vi "CRYCalc FSD.vi"(10 "Max Level":dbl format="%#_6p", 11 "X":dbl[](array[numeric]) format="%.2p") -> (0 "dBFSD(RMS)":dbl format="%#_6p", 1 "%FSD(RMS)":dbl format="%#_6p", 2 "dBFSD(Max)":dbl format="%#_6p", 3 "%FSD(Max)":dbl format="%#_6p")   [LabVIEW 2013]
uses:
  <vilib>/Analysis/5stat.llb/RMS (DBL).vi
  <vilib>/Analysis/NI_AALPro.lvlib
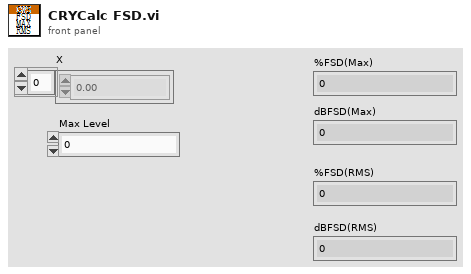
[diagram p1: front panel]
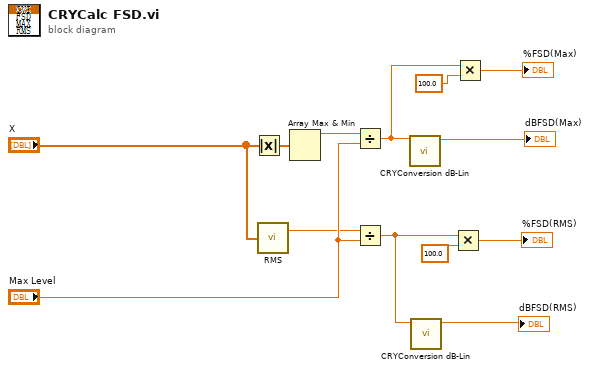
[diagram p0: block diagram]
diagram:
  n1 = Absolute Value(x="X") -> (abs(x)=w12:dbl[])
  n2 = call-poly <vilib>:"RMS.vi"("X"="X") -> ("rms value"=w3:dbl)  [unwired: 1 out]
  n3 = Array Max & Min(array=w12) -> (max value=w5:dbl)  [unwired: 3 out]
  n4 = Divide(x=w5, y="Max Level") -> (x/y=w7:dbl)
  n5 = Divide(x=w3, y="Max Level") -> (x/y=w2:dbl)
  n6 = call "CRYConversion dB-Lin.vi"("Lin In"=w7) -> ("Log Out"=→"dBFSD(Max)":dbl)  [unwired: 5 in, 3 out]
  n7 = call "CRYConversion dB-Lin.vi"("Lin In"=w2) -> ("Log Out"=→"dBFSD(RMS)":dbl)  [unwired: 5 in, 3 out]
  n8 = Multiply(x=w2, y=100.0) -> (x*y=→"%FSD(RMS)":dbl)
  n9 = Multiply(x=w7, y=100.0) -> (x*y=→"%FSD(Max)":dbl)
